vi "mWmotor_rev_to_freq.vi"(9 "Intercept":dbl, 10 "Slope":dbl, 11 "Revolution":dbl) -> (3 "Frequecy":dbl)   [LabVIEW 2019]
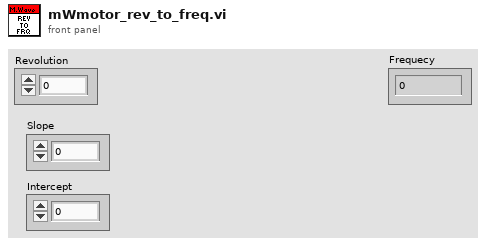
[diagram p1: front panel]
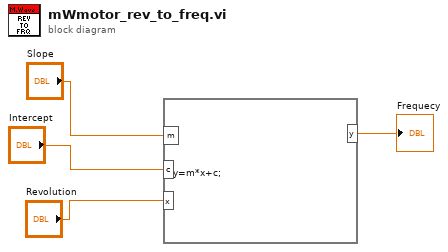
[diagram p0: block diagram]
diagram:
  n1 = formula code="y=m*x+c;"("m"="Slope", "c"="Intercept", "x"="Revolution") -> ("y"=→"Frequecy":dbl)
